vi "Create Data1D.vi"(8 "error in (no error)":errorcluster, 10 "dt":dbl format="%#_13g", 11 "Array":dbl[](array[numeric])) -> (0 "error out":errorcluster, 3 "Data1D out":refnum<class "Data1D.lvclass">)   [LabVIEW 2014, in "Data1D.lvclass"]
uses:
  Data1D.lvclass
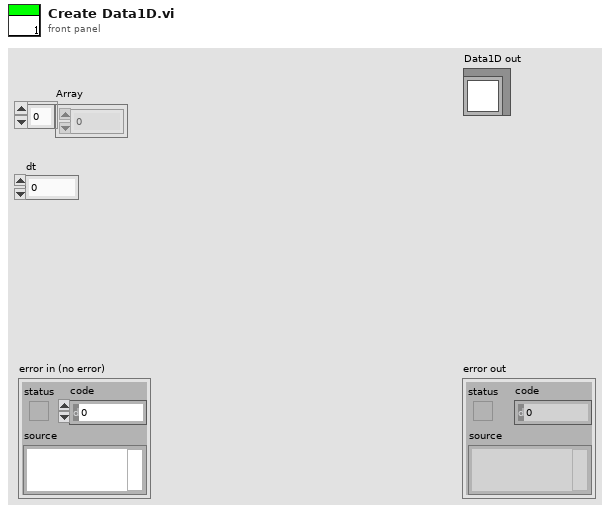
[diagram p1: front panel]
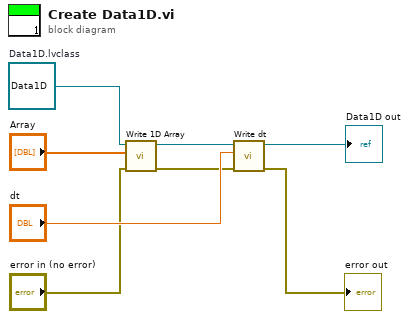
[diagram p0: block diagram]
diagram:
  w4 = refnum<class "Data1D.lvclass"> refnum  # Data1D.lvclass
  n1 = call "Write 1D Array.vi"("error in (no error)"="error in (no error)", "1D Array"="Array", "Data1D in"=w4) -> ("error out"=w5:errorcluster, "Data1D out"=w6:refnum<class "Data1D.lvclass">)  [unwired: 7 in]
  n2 = call "Write dt.vi"("error in (no error)"=w5, "dt"="dt", "Data1D in"=w6) -> ("error out"=→"error out":errorcluster, "Data1D out"=→"Data1D out":refnum<class "Data1D.lvclass">)  [unwired: 7 in]
